vi "Verify Key Match.vi"(8 "error in (no error)":errorcluster, 10 "Shared Key":string, 11 "Attribute.Owner in":refnum<class "Attribute.Owner.lvclass">) -> (0 "error out":errorcluster, 2 "key matched":bool, 3 "Attribute.Owner out":refnum<class "Attribute.Owner.lvclass">)   [LabVIEW 2013, in "Attribute.Owner.lvclass"]
uses:
  Attribute.Owner.lvclass
  Attribute.Owner.lvclass/Attribute.Owner.ctl
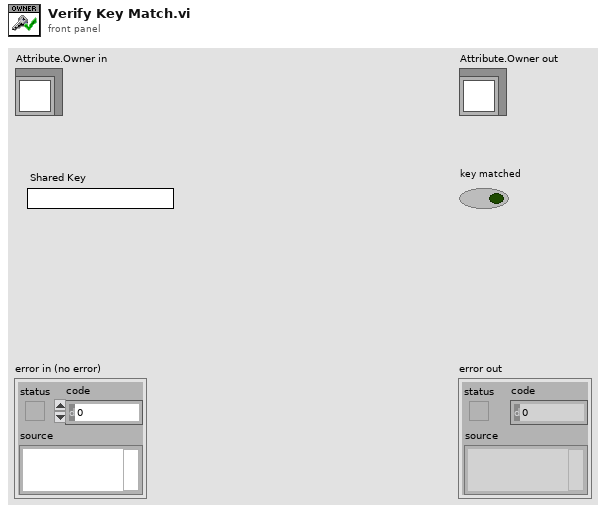
[diagram p1: front panel]
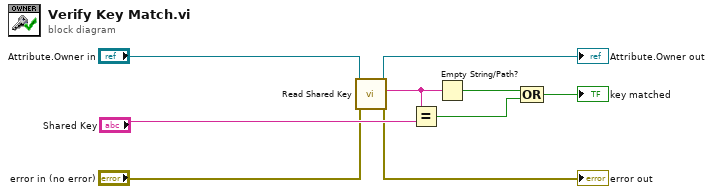
[diagram p0: block diagram]
diagram:
  n1 = call "Read Shared Key.vi"("error in (no error)"="error in (no error)", "Attribute.Owner in"="Attribute.Owner in") -> ("error out"=→"error out":errorcluster, "Shared Key"=w4:string, "Attribute.Owner out"=→"Attribute.Owner out":refnum<class "Attribute.Owner.lvclass">)  [unwired: 7 in]
  n2 = Equal?(x=w4, y="Shared Key") -> (x = y?=w2:bool)
  n3 = Empty String/Path?(string/path=w4) -> (empty?=w3:bool)
  n4 = Compound Arithmetic op=OR(w3, w2) -> (→"key matched":bool)
